vi "Test Pump Control.vi"() -> ()   [LabVIEW 2024]
uses:
  Control Definitions/Def FullCfg.ctl
  Control Definitions/Def BenchCfg.ctl
  Control Definitions/Def PumpCtlRefs.ctl
  Control Definitions/Def Bench Status.ctl
panel:
  out "TEST STATUS Out":T1(ring)=enum."Done"
  in  "Full Config":T2={"Bench Config"={"Name"="OLR001", {"Step Levels"=0.05, "Tolerance"=0.01, "Sample Rate"=0.05, "Resistor"=100.0, "M Level Cal"=1.0, "[B Level Cal"=0.0, "Max Fill Rate"=0.025, "Max Gal"=10.0, "Max Inches"=10.0}}, "Test Value Table "=[[0.0, 0.0, 0.0, 0.0, 0.0, 0.0, 0.0, 0.0, 0.0, 0.0], [100.0, 2.0, 7.91, 8.01, 7.55, 7.65, 7.685, 7.785, 7.325, 7.425], [200.0, 3.0, 7.46, 7.56, 7.1, 7.2, 7.235, 7.335, 6.875, 6.975], [300.0, 4.0, 7.01, 7.11, 6.65, 6.75, 6.785, 6.885, 6.425, 6.525], [400.0, 5.0, 6.56, 6.66, 6.2, 6.3, 6.335, 6.435, 5.975, 6.075], [500.0, 6.0, 6.11, 6.21, 5.75, 5.85, 5.885, 5.985, 5.525, 5.625], [600.0, 7.0, 5.66, 5.76, 5.3, 5.4, 5.435, 5.535, 5.075, 5.175], [700.0, 8.0, 5.21, 5.31, 4.85, 4.95, 4.985, 5.085, 4.625, 4.725], [800.0, 9.0, 4.76, 4.86, 4.4, 4.5, 4.535, 4.635, 4.175, 4.275], [900.0, 10.0, 4.31, 4.41, 3.95, 4.05, 4.085, 4.185, 3.725, 3.825], [1000.0, 11.0, 3.86, 3.96, 3.5, 3.6, 3.635, 3.735, 3.275, 3.375], [1100.0, 12.0, 3.41, 3.51, 3.05, 3.15, 3.185, 3.285, 2.825, 2.925]], "Table Col Titles"=[["A Resist", "A Tolerence", "A Fill Lo", "A Fill Hi", "A Drain Lo", "A Drain Hi", "B Fill Lo", "B Fill Hi", "B Drain Lo", "B Drain Hi"]], "Pump CtlRef In"={"Fill "=refnum, "Drain"=refnum, "Level PV"=refnum, "Flow Rate%"=refnum, "Run Test"=refnum, "Sim"=refnum, "Jog"=refnum, "Level SP"=refnum}, "Bench Status"={"Pump Status"=refnum, "Instrumnet\n Status"=refnum}}
  out "Fill Out":bool=TRUE
  out "Drain Out":bool
  in  "stop":bool
  in  "Level SP":dbl(slide)=2.142857142857143 scale=0.0..10.0
  in  "Flow Rate %":dbl(knob)=100.0 scale=0.0..100.0
  in  "Pump JOG":bool
  in  "Run Test":bool
  in  "Simulate":bool
  in  "Drain":bool
  in  "Fill":bool=TRUE
  in  "Level PV":dbl(slide) scale=0.0..10.0
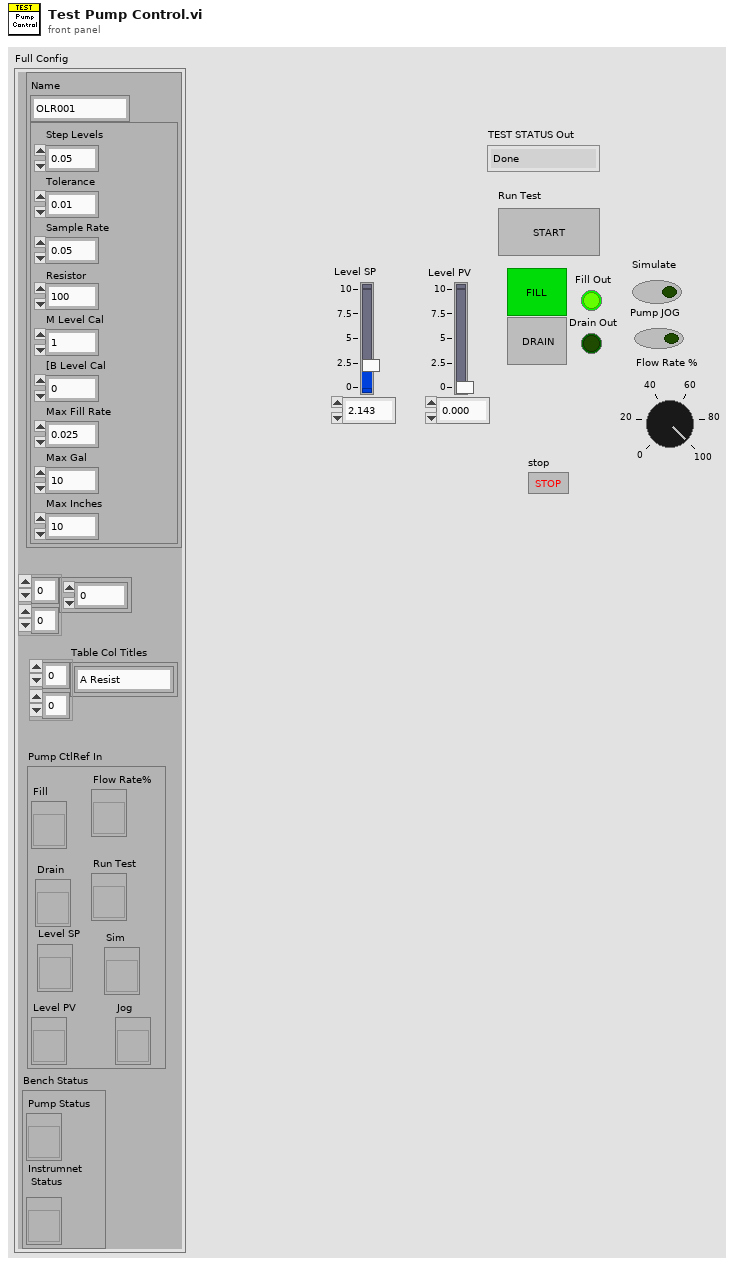
[diagram p1: front panel]
types:
  T1 = enum16{"MANUAL", "Start", "Filling", "FULL", "Draining", "EMPTY", "Done"}
  T2 = typedef "Def FullCfg.ctl" = cluster{"Bench Config":T3, "Test Value Table ":dbl[][], "Table Col Titles":string[][], "Pump CtlRef In":T4, "Bench Status":T5}
  T3 = typedef "Def BenchCfg.ctl" = cluster{"Name":string, cluster{"Step Levels":dbl, "Tolerance":dbl, "Sample Rate":dbl, "Resistor":dbl, "M Level Cal":dbl, "[B Level Cal":dbl, "Max Fill Rate":dbl, "Max Gal":dbl, "Max Inches":dbl}}
  T4 = typedef "Def PumpCtlRefs.ctl" = cluster{"Fill ":refnum<vi>, "Drain":refnum<vi>, "Level PV":refnum<vi>, "Flow Rate%":refnum<vi>, "Run Test":refnum<vi>, "Sim":refnum<vi>, "Jog":refnum<vi>, "Level SP":refnum<vi>}
  T5 = typedef "Def Bench Status.ctl" = cluster{"Pump Status":refnum<vi>, "Instrumnet\n Status":refnum<vi>}
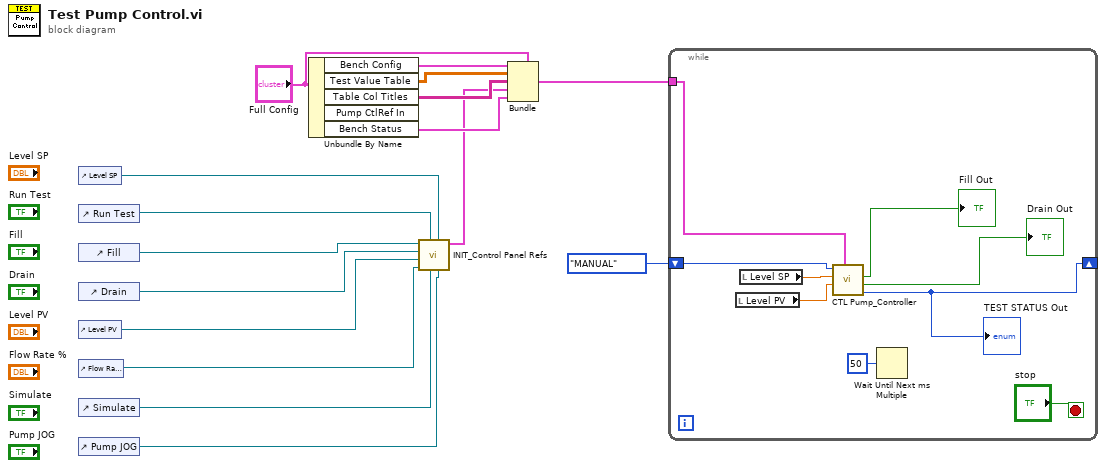
[diagram p0: block diagram]
diagram:
  n1 = control-ref of="Level SP"() -> (w9:refnum<vi>)
  n2 = control-ref of="Run Test"() -> (w16:refnum<vi>)
  n3 = control-ref of="Fill"() -> (w15:refnum<vi>)
  n4 = control-ref of="Drain"() -> (w14:refnum<vi>)
  n5 = control-ref of="Level PV"() -> (w12:refnum<vi>)
  n6 = control-ref of="Flow Rate %"() -> (w13:refnum<vi>)
  n7 = control-ref of="Simulate"() -> (w11:refnum<vi>)
  n8 = control-ref of="Pump JOG"() -> (w10:refnum<vi>)
  n9 = Unbundle By Name("Full Config") -> ("Bench Config"=w8:T3, "Test Value Table"=w7:dbl[][], "Table Col Titles"=w5:string[][], "Bench Status"=w4:T5)  [unwired: 1 out]
  n10 = call "INIT_Control Panel Refs.vi"("Jog"=w10, "Level SP"=w9, "Sim"=w11, "Run Test"=w16, "Flow Rate %"=w13, "Level PV"=w12, "Drain"=w14, "Fill"=w15) -> ("PumpCtlRef out"=w3:T4)  [unwired: 3 in]
  n11 = Bundle(cluster="Full Config", "Bench Config"=w8, "Test Value Table"=w7, "Table Col Titles"=w5, "Pump CtlRef In"=w3, "Bench Status"=w4) -> (w2:T2)
  n12 = while {
    tunnel: w2 -> [w24]
    shift-right: [w17] -> _
    shift-left: T1."MANUAL" ("TEST STATUS In") -> [w18]
    stop <- "stop" stop-if-true
    n13 = local read "Level PV"() -> (w20:dbl)
    n14 = local read "Level SP"() -> (w21:dbl)
    n15 = call "CTL Pump_Controller.vi"("Full Config"=w24, "Level PV"=w20, "Level SP"=w21, "TEST State In"=w18) -> ("TEST State Out"=w17:T1, "Drain Out"=→"Drain Out":bool, "Fill Out"=→"Fill Out":bool)  [unwired: 4 in, 1 out]
    "TEST STATUS Out" <- w17
    n16 = Wait Until Next ms Multiple(millisecond multiple=u32 50) -> ()  [unwired: 1 out]
  }
